vi "1.3.17 New Lidar Transfer.vi"   [LabVIEW 2010]
uses:
  <vilib>/rvi/DataTransferAndStorage/Container/XNode/niFpgaContainer.xnode
  <vilib>/rvi/DataTransferAndStorage/Container/Common/niFpgaContainerMethod.ctl
  <vilib>/rvi/DataTransferAndStorage/Container/Common/niFpgaTransferTypeControl.ctl
  <vilib>/rvi/FIFO/Fifo_Resource/nirvififoEmulationSetSize.vi
  <vilib>/rvi/DataTransferAndStorage/Container/Common/niFpgaContainerGetUniqueNameForEmu.vi
  1.0-Hindbrain Global.vi
  Lidar Test Global.vi
  <vilib>/rvi/interface/RandomDataEmulation/nirviRandomDataFPGAFIFO.vi
  <vilib>/rvi/interface/RandomDataEmulation/niFpgaRandomDataHandleErrors.vi
types:
  T1 = enum16{"confirm check sum", "check status byte", "read measured values", "confirm measurement", "confirm command", "read message length", "read address", "wait for \"02\""}
  T2 = typedef "niFpgaContainerMethod.ctl" = enum16{"<none>", "write", "read", "clear", "getNumberOfElementsToWrite", "getNumberOfElementsToRead", "enable", "disable", "flushAndDisable", "getStreamState", "readA", "readB", "dramWrite", "dramWriteWithByteEnables", "dramRequestData", "dramRetrieveData"}
  T3 = typedef "niFpgaTransferTypeControl.ctl" = enum16{"Target-Scoped", "Host to Target - DMA", "Target to Host - DMA", "Peer to Peer Reader", "Peer to Peer Writer", "Bidirectional"}
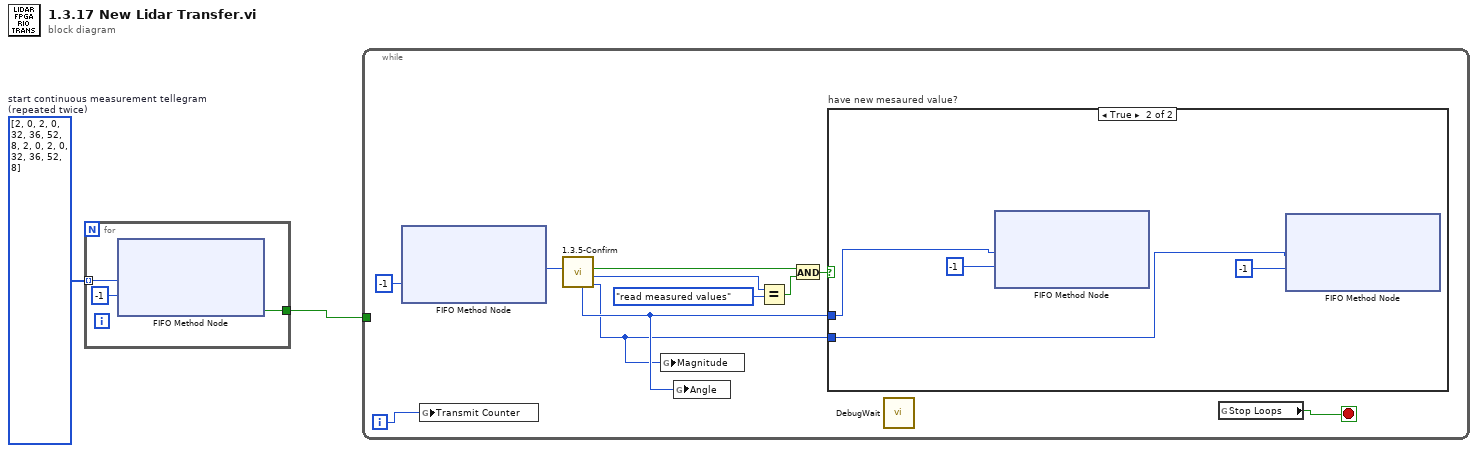
[diagram p0: block diagram]
diagram:
  w1 = u8[] [2, 0, 2, 0, 32, 36, 52, 8, 2, 0, 2, 0, 32, 36, 52, 8]  # start continuous measurement tellegram (repeated twice)
  n1 = for {
    tunnel: w1 -> [w5] mode=indexing
    tunnel: [w3] -> w2
    n2 = xnode ("FIFO Method Node")("Element"=w5, "Timeout"=-1) -> ("Timed Out?"=w3:bool)  [unwired: 1 in, 1 out]
  }
  n3 = while {
    tunnel: w2 -> [_]
    i -> [w57]
    stop <- w60 stop-if-true
    n4 = xnode ("FIFO Method Node")("Timeout"=-1) -> ("Element"=w67:u8)  [unwired: 1 in, 2 out]
    n5 = global write "Lidar Test Global.vi" "Transmit Counter"(w57) -> ()
    n6 = call "1.3.5-Confirm.vi"("LIDAR raw data"=w67) -> ("last measured value"=w58:u16, "parser state"=w66:T1, "new value?"=w65:bool, "angle"=w59:u8)  [unwired: 7 in]
    n7 = global write "Lidar Test Global.vi" "Magnitude"(w58) -> ()
    n8 = global write "Lidar Test Global.vi" "Angle"(w59) -> ()
    n9 = Equal?(x=w66, y=T1."read measured values" ("parser state")) -> (x = y?=w62:bool)
    n10 = And(x=w65, y=w62) -> (x .and. y?=w64:bool)
    n11 = case "have new mesaured value?" shown="True" w64 {
      tunnel: w58 -> [_ w122]
      tunnel: w59 -> [_ w120]
      frame False {
      }
      frame True {
        n12 = xnode ("FIFO Method Node")("Element"=w120, "Timeout"=-1) -> ()  [unwired: 1 in, 2 out]
        n13 = xnode ("FIFO Method Node")("Element"=w122, "Timeout"=-1) -> ()  [unwired: 1 in, 2 out]
      }
    }
    n14 = call "DebugWait.vi"() -> ()  [unwired: 12 in]
    n15 = global read "1.0-Hindbrain Global.vi" "Stop Loops"() -> (w60:bool)
  }
